vi "Signal Timer test.vi"() -> ()   [LabVIEW 2013]
panel:
  in  "Edge":bool
  in  "Interval":dbl format="%#_13g"
  out "Filtered Output":bool
  in  "Pull Up (T)?":bool=TRUE
  in  "Input":bool
  in  "stop":bool
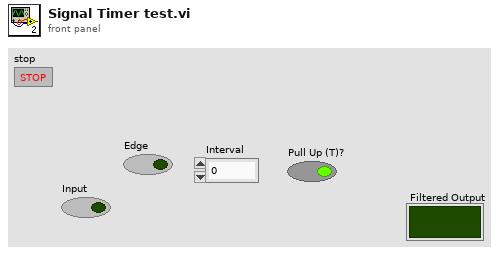
[diagram p1: front panel]
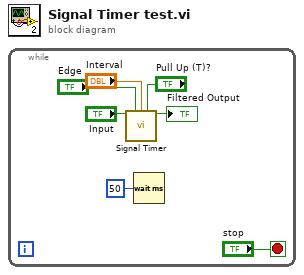
[diagram p0: block diagram]
diagram:
  n1 = while {
    stop <- "stop" stop-if-true
    n2 = call "Signal Timer.vi"("Input"="Input", "Edge"="Edge", "Interval"="Interval", "Pull"="Pull Up (T)?") -> ("Filtered Output"=→"Filtered Output":bool)  [unwired: 11 in]
    n3 = Wait (ms)(milliseconds to wait=u32 50) -> ()  [unwired: 1 out]
  }
